vi "FT10_Date and Time String.vi"(9 "Include msec":bool, 11 "to UTC":bool) -> (3 "Date & Time string":string)   [LabVIEW 2015]
doc: "Converts current date and time to string.\n\nUTC = Coordinated Universal Time"
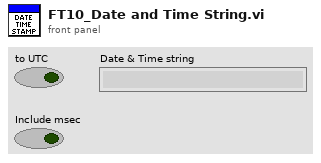
[diagram p1: front panel]
types:
  T1 = typedef "LVDateTimeRec.ctl" = cluster{"fractional second":dbl, "second":i32, "minute":i32, "hour":i32, "day of month":i32, "month":i32, "year":i32, "day of week":i32, "day of year":i32, "DST":i32}
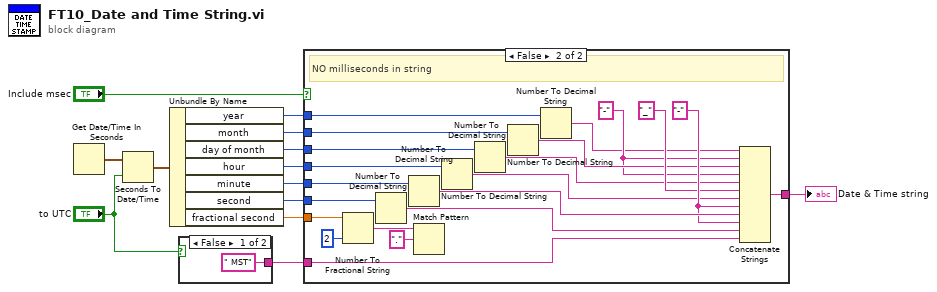
[diagram p0: block diagram]
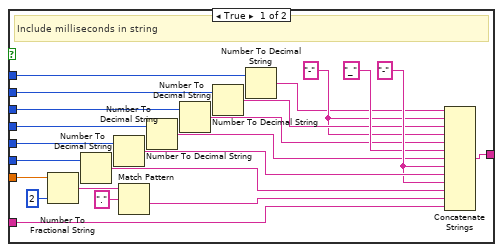
[diagram p2: hidden frame]
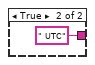
[diagram p3: hidden frame]
diagram:
  n1 = Get Date/Time In Seconds() -> (seconds since 1Jan1904=w3:timestamp)
  n2 = Seconds To Date/Time(time stamp (now)=w3, to UTC (F)="to UTC") -> (date time rec=w4:T1)
  n3 = Unbundle By Name(w4) -> ("year"=w5:i32, "month"=w6:i32, "day of month"=w7:i32, "hour"=w8:i32, "minute"=w9:i32, "second"=w10:i32, "fractional second"=w2:dbl)
  n4 = case shown="False" "to UTC" {
    tunnel: [" MST" ("string") " UTC" ("string")] -> w13
    frame False {
    }
    frame True {
    }
  }
  n5 = case shown="False" "Include msec" {
    tunnel: w13 -> [w17 w58]
    tunnel: [w29 w49] -> w11
    tunnel: w10 -> [w28 w48]
    tunnel: w9 -> [w27 w47]
    tunnel: w8 -> [w26 w46]
    tunnel: w7 -> [w25 w45]
    tunnel: w6 -> [w24 w44]
    tunnel: w5 -> [w23 w43]
    tunnel: w2 -> [w22 w42]
    frame True {
      w36 = "-" ("string")
      w31 = "-" ("string")
      # "Include milliseconds in string"
      n6 = Number To Fractional String(number=w22, precision (6)=i16 2) -> (F-format string=w21:string)  [unwired: 2 in]
      n7 = Number To Decimal String(number=w28) -> (decimal integer string=w20:string)  [unwired: 1 in]
      n8 = Number To Decimal String(number=w27) -> (decimal integer string=w37:string)  [unwired: 1 in]
      n9 = Match Pattern(string=w21, regular expression=".") -> (after substring=w16:string)  [unwired: 1 in, 3 out]
      n10 = Number To Decimal String(number=w26) -> (decimal integer string=w35:string)  [unwired: 1 in]
      n11 = Number To Decimal String(number=w25) -> (decimal integer string=w33:string)  [unwired: 1 in]
      n12 = Number To Decimal String(number=w24) -> (decimal integer string=w32:string)  [unwired: 1 in]
      n13 = Number To Decimal String(number=w23) -> (decimal integer string=w30:string)  [unwired: 1 in]
      n14 = Concatenate Strings(w30, w31, w32, w31, w33, "_" ("string"), w35, w36, w37, w36, w20, w16, w17) -> (w29:string)
    }
    frame False {
      w56 = "-" ("string")
      w51 = "-" ("string")
      # "NO milliseconds in string"
      n15 = Number To Fractional String(number=w42, precision (6)=i16 2) -> (F-format string=w41:string)  [unwired: 2 in]
      n16 = Number To Decimal String(number=w48) -> (decimal integer string=w40:string)  [unwired: 1 in]
      n17 = Number To Decimal String(number=w47) -> (decimal integer string=w57:string)  [unwired: 1 in]
      n18 = Match Pattern(string=w41, regular expression=".") -> ()  [unwired: 1 in, 4 out]
      n19 = Number To Decimal String(number=w46) -> (decimal integer string=w55:string)  [unwired: 1 in]
      n20 = Number To Decimal String(number=w45) -> (decimal integer string=w53:string)  [unwired: 1 in]
      n21 = Number To Decimal String(number=w44) -> (decimal integer string=w52:string)  [unwired: 1 in]
      n22 = Number To Decimal String(number=w43) -> (decimal integer string=w50:string)  [unwired: 1 in]
      n23 = Concatenate Strings(w50, w51, w52, w51, w53, "_" ("string"), w55, w56, w57, w56, w40, w58) -> (w49:string)
    }
  }
  "Date & Time string" <- w11
